vi "beta-1.0.0.vi"() -> ()   [LabVIEW 2016]
uses:
  <vilib>/FPGAPlugInAG/cRIO-9063/niLvFpga_Open_cRIO-9063.vi
  <vilib>/rvi/interface/common/dynamic/niFpgaDynamicAddResources.vi
  <vilib>/Utility/error.llb/Error Cluster From Error Code.vi
  <vilib>/rvi/errors/niLvFpgaAdjustHostInterfaceError.vi
  <vilib>/FPGAPlugInAG/Dynamic/niLvFpga_Close_Dynamic.vi
  <vilib>/rvi/interface/nirviOpenFPGA/nirviOpenFPGA.xnode
  FPGA Bitfiles/multi-functionpr_FPGATarget_DI&AO_PaHU11gpxn0.lvbitx
  DI&AO.vi
  <vilib>/rvi/interface/nirviReadWriteControl/nirviReadWriteControl.xnode
  <vilib>/rvi/interface/nirviCloseFPGA/nirviCloseFPGA.xnode
  NiFpgaLv.dll
  <vilib>/rvi/interface/Simulation/niFpgaSimulationCallBeginRW.vi
panel:
  out "Mod2/DIO3":bool
  out "Mod2/DIO2":bool
  in  "end1":dbl=5.0 format="%#_13g"
  in  "begin1":dbl format="%#_13g"
  in  "step1":dbl=1.0 format="%#_13g"
  in  "OUT1":T1(ring)
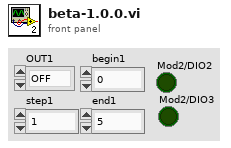
[diagram p1: front panel]
types:
  T1 = enum16{"OFF", "SWITCH", "AND GATE", "OR GATE", "ITERATION"}
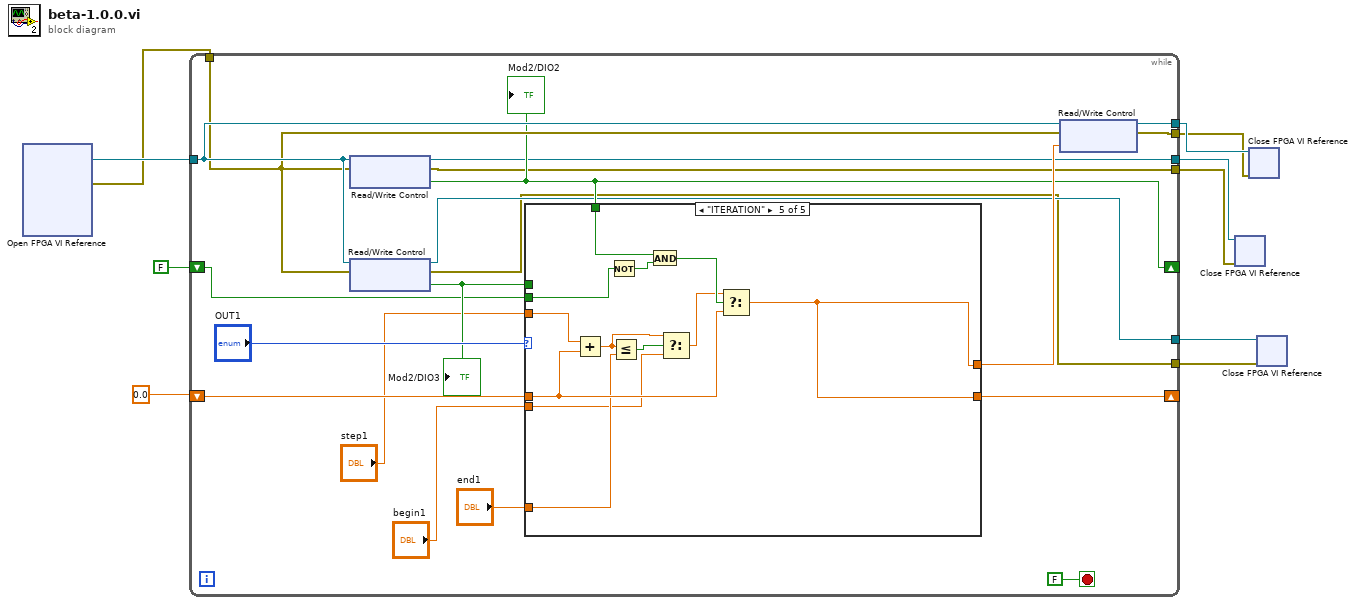
[diagram p0: block diagram]
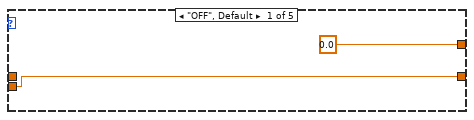
[diagram p2: hidden frame]
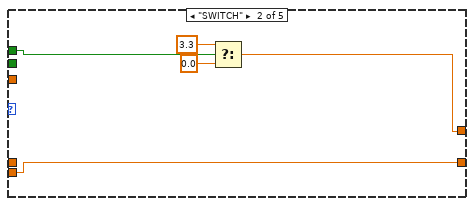
[diagram p3: hidden frame]
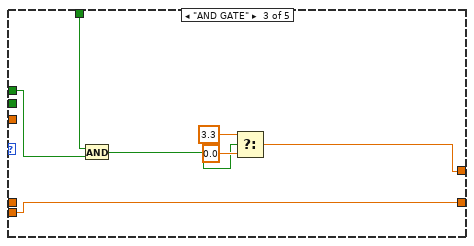
[diagram p4: hidden frame]
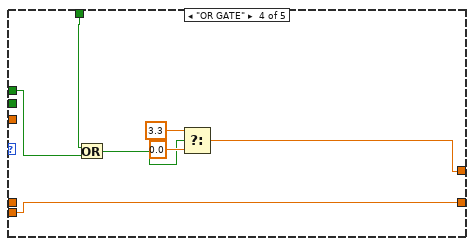
[diagram p5: hidden frame]
diagram:
  n1 = xnode "Open FPGA VI Reference"() -> ("FPGA VI Reference Out"=w10:refnum<k20>, "error out"=w1:errorcluster)  [unwired: 2 in]
  n2 = while {
    tunnel: w10 -> [w27]
    tunnel: w1 -> [w26]
    shift-right: [w19] -> _
    shift-left: 0.0 -> [w21]
    shift-right: [w23] -> _
    shift-left: FALSE -> [w22]
    tunnel: [w16] -> w7
    tunnel: [w15] -> w6
    tunnel: [w14] -> w5
    tunnel: [w13] -> w4
    tunnel: [w12] -> w3
    tunnel: [w11] -> w2
    stop <- FALSE stop-if-true
    n3 = xnode "Read/Write Control"("FPGA VI Reference In"=w27, "error in"=w26) -> ("FPGA VI Reference Out"=w14:refnum<k20>, "error out"=w13:errorcluster, "Mod2/DIO2"=w23:bool)
    "Mod2/DIO2" <- w23
    n4 = xnode "Read/Write Control"("FPGA VI Reference In"=w27, "error in"=w26) -> ("FPGA VI Reference Out"=w16:refnum<k20>, "error out"=w15:errorcluster, "Mod2/DIO3"=w25:bool)
    "Mod2/DIO3" <- w25
    n5 = case shown="\"ITERATION\"" "OUT1" {
      tunnel: w25 -> [_ w36 w42 w49 _]
      tunnel: [0.0 w33 w38 w45 w57] -> w24
      tunnel: w23 -> [_ _ w43 w50 w60]
      tunnel: w22 -> [_ _ _ _ w62]
      tunnel: w21 -> [_ _ _ _ w56]
      tunnel: "step1" -> [_ _ _ _ w58]
      tunnel: [w30 w32 w37 w44 w57] -> w19
      tunnel: "begin1" -> [w30 w32 w37 w44 w52]
      tunnel: "end1" -> [_ _ _ _ w55]
      frame "OFF", Default {
      }
      frame "SWITCH" {
        n6 = Select(t=3.3, s=w36, f=0.0) -> (s? t:f=w33:dbl)
      }
      frame "AND GATE" {
        n7 = And(x=w43, y=w42) -> (x .and. y?=w39:bool)
        n8 = Select(t=3.3, s=w39, f=0.0) -> (s? t:f=w38:dbl)
      }
      frame "OR GATE" {
        n9 = Or(x=w50, y=w49) -> (x .or. y?=w46:bool)
        n10 = Select(t=3.3, s=w46, f=0.0) -> (s? t:f=w45:dbl)
      }
      frame "ITERATION" {
        n11 = Add(x=w58, y=w56) -> (x+y=w53:dbl)
        n12 = Not(x=w62) -> (.not. x?=w61:bool)
        n13 = Less Or Equal?(x=w53, y=w55) -> (x <= y?=w54:bool)
        n14 = And(x=w60, y=w61) -> (x .and. y?=w59:bool)
        n15 = Select(t=w53, s=w54, f=w52) -> (s? t:f=w51:dbl)
        n16 = Select(t=w51, s=w59, f=w56) -> (s? t:f=w57:dbl)
      }
    }
    n17 = xnode "Read/Write Control"("FPGA VI Reference In"=w27, "error in"=w26, "Mod4/AO1"=w24) -> ("FPGA VI Reference Out"=w12:refnum<k20>, "error out"=w11:errorcluster)
  }
  n18 = xnode "Close FPGA VI Reference"("FPGA VI Reference In"=w5, "error in"=w4) -> ()  [unwired: 1 out]
  n19 = xnode "Close FPGA VI Reference"("FPGA VI Reference In"=w3, "error in"=w2) -> ()  [unwired: 1 out]
  n20 = xnode "Close FPGA VI Reference"("FPGA VI Reference In"=w7, "error in"=w6) -> ()  [unwired: 1 out]
